vi "Save-Load-Edit ESP Table.vi"(0 "ESP Table Cluster":refnum<vi>, 5 "Table Folder":path, 11 "ESP Table Cluster":T1={"ON-DEMAND Config"=FALSE, "ON-DEMAND Active Commands"=[27, 28, 29], "CONTINUOUS Config"=FALSE, "CONTINUOUS Active Commands"=[41], "ERROR Config"=FALSE, "ERROR Command"="38", "STATUS Config"=FALSE, "STATUS Command"="37", "DIGITAL Config"=FALSE, "DIGITAL Command"="39", "SAVE TABLE"=FALSE, "Active Table"=0, "New Table Name"="38", "NEW CMD TABLE"=[36]} {"Active Table" items=["123", "a", "b", "c"]}, 12 "ENABLE":bool=TRUE) -> (15 "Error Output":errorcluster)   [LabVIEW 2011]
panel:
  # "SAVE - LOAD - EDIT \nESP Command Table"
  # "Blake Otting - Ecolab\nCreated 7-11-2012"
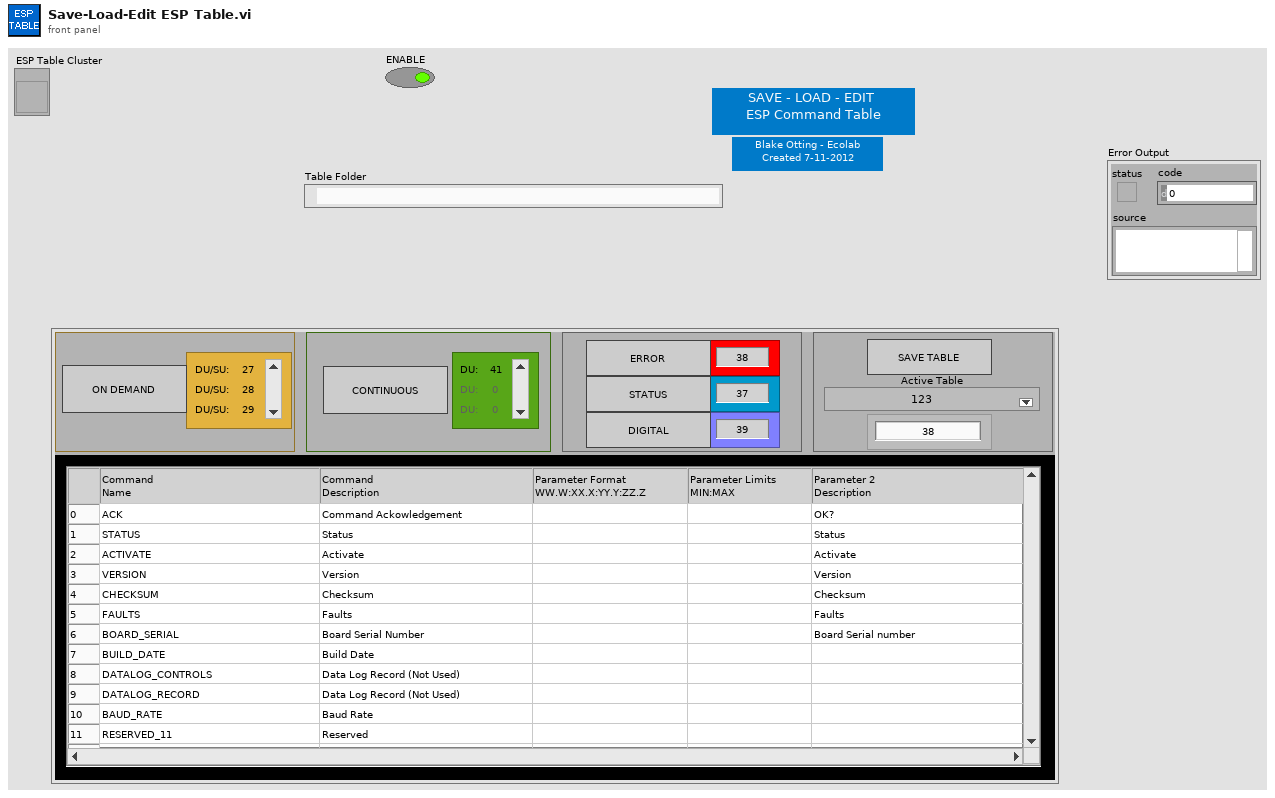
[diagram p1: front panel]
types:
  T1 = cluster{"ON-DEMAND Config":bool, "ON-DEMAND Active Commands":i32[], "CONTINUOUS Config":bool, "CONTINUOUS Active Commands":i32[], "ERROR Config":bool, "ERROR Command":string, "STATUS Config":bool, "STATUS Command":string, "DIGITAL Config":bool, "DIGITAL Command":string, "SAVE TABLE":bool, "Active Table":u16, "New Table Name":string, "NEW CMD TABLE":i32[]}
  T2 = cluster{"ON Demand Button":i32, "ON Demand Commands":i32, "Continuous Button":i32, "Continuous Commands":i32, "Error Button":i32, "Error Command":i32, "Status Button":i32, "Status Command":i32, "Digital Button":i32, "Digital Command":i32, "Save Table Button":i32, "Active Table":i32, "New Table Name":i32, "Table":i32}
  T3 = enum8{"Enabled", "Disabled", "Disabled and Grayed Out"}
  T4 = enum16{"open", "replace", "create", "open or create", "replace or create", "replace or create with confirmation"}
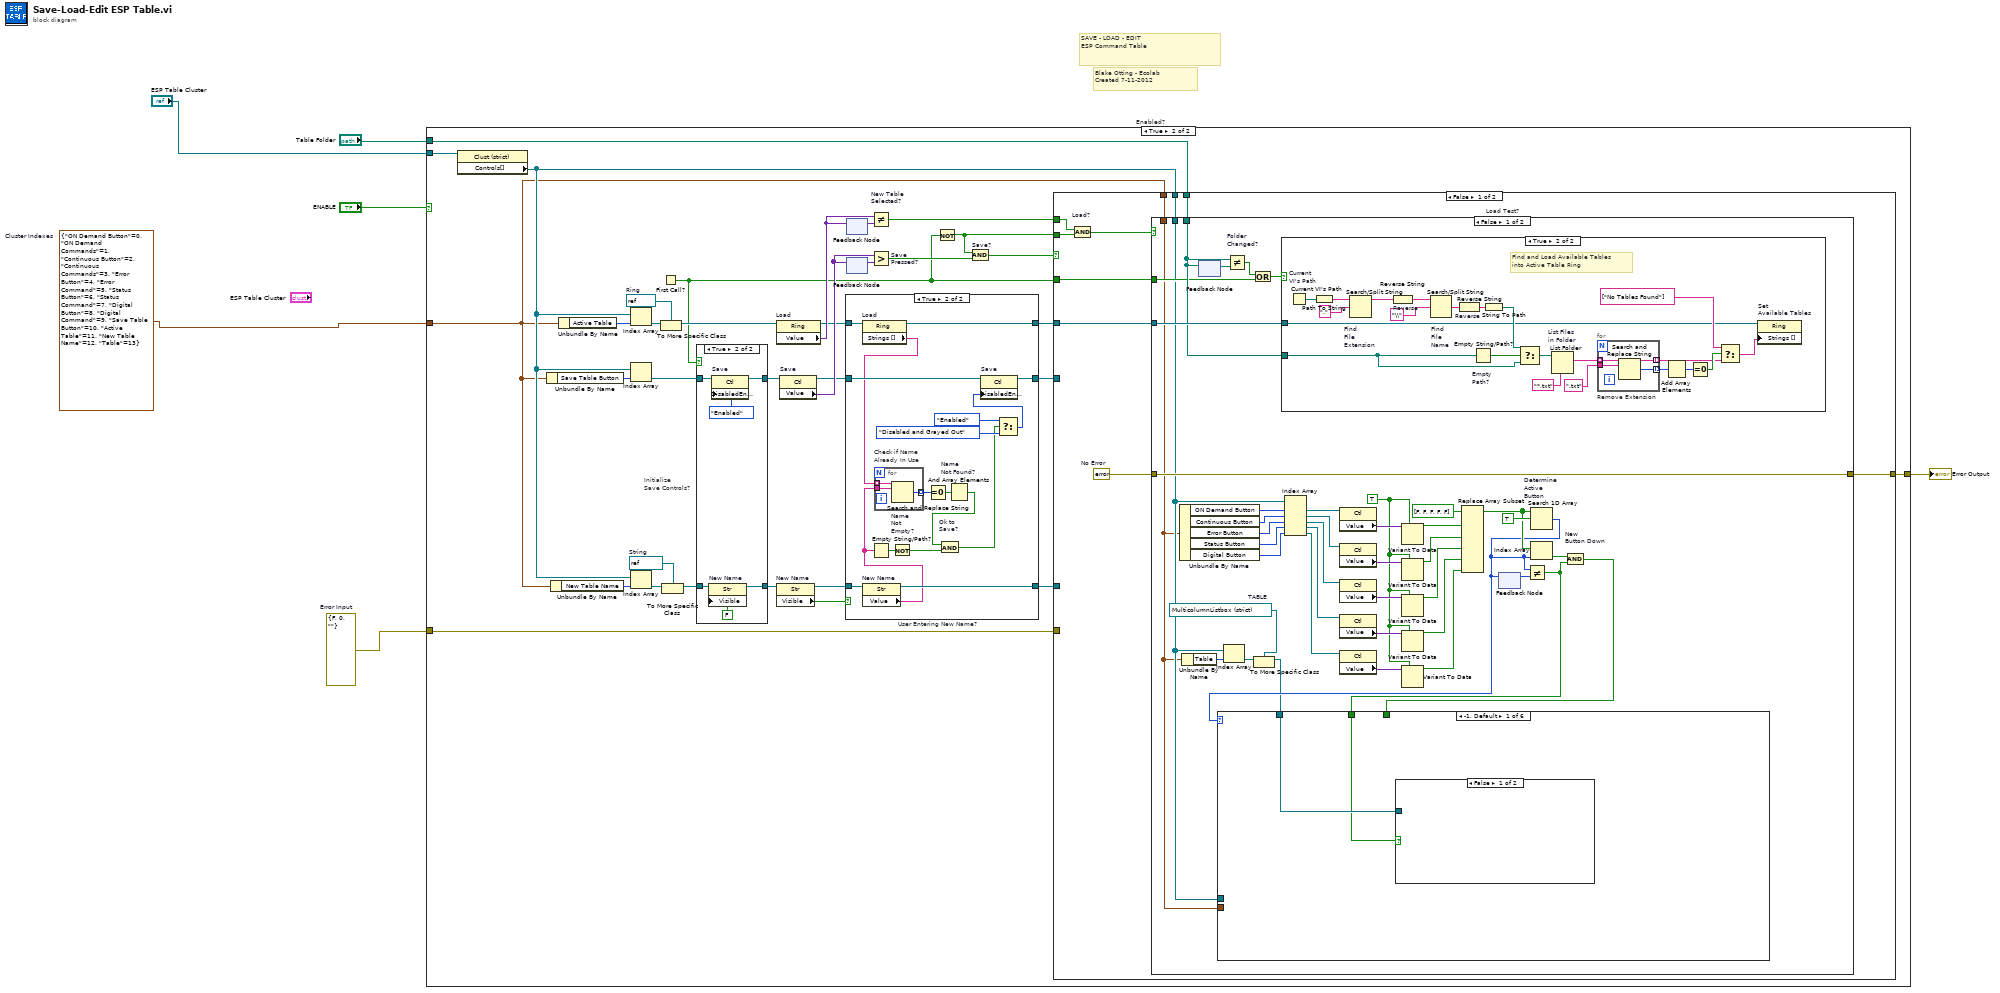
[diagram p0: block diagram]
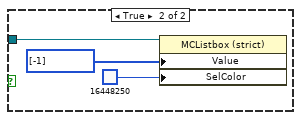
[diagram p5: hidden frame]
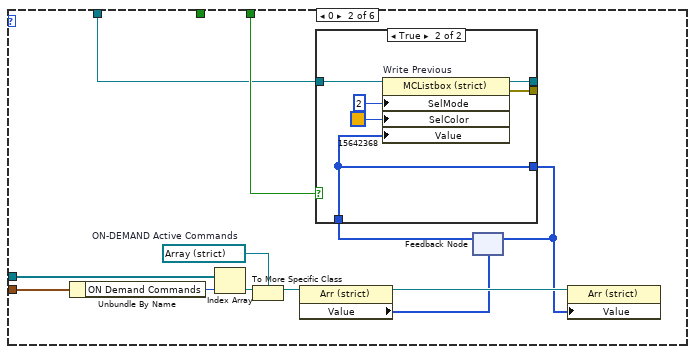
[diagram p6: hidden frame]
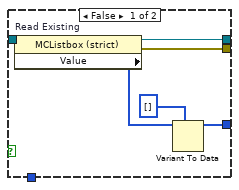
[diagram p7: hidden frame]
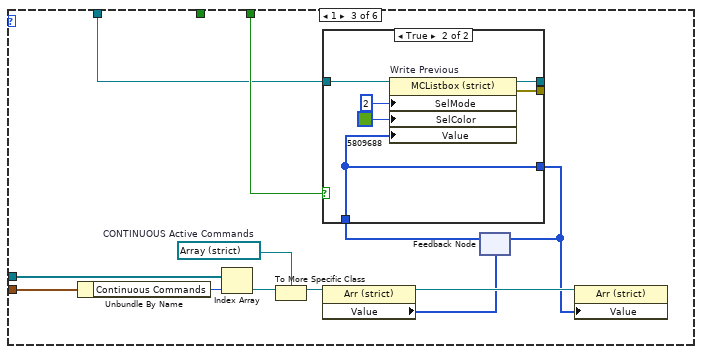
[diagram p8: hidden frame]
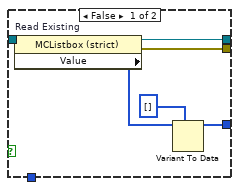
[diagram p9: hidden frame]
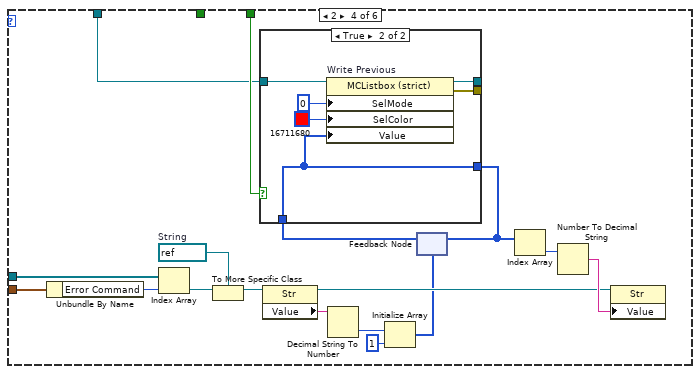
[diagram p10: hidden frame]
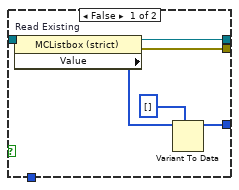
[diagram p11: hidden frame]
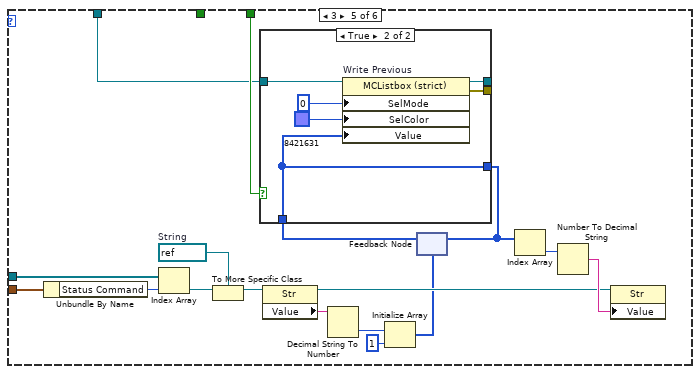
[diagram p12: hidden frame]
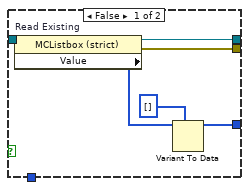
[diagram p13: hidden frame]
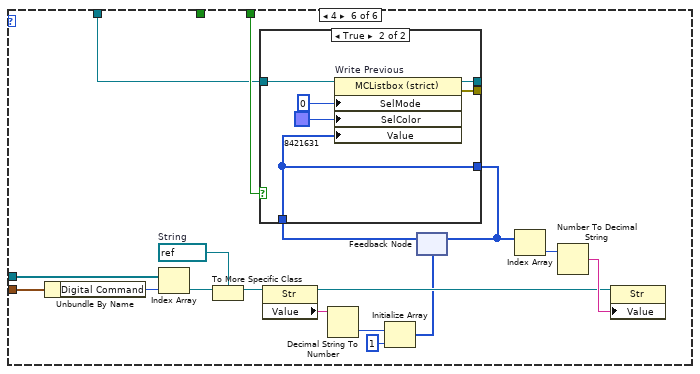
[diagram p14: hidden frame]
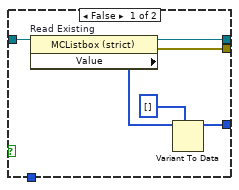
[diagram p15: hidden frame]
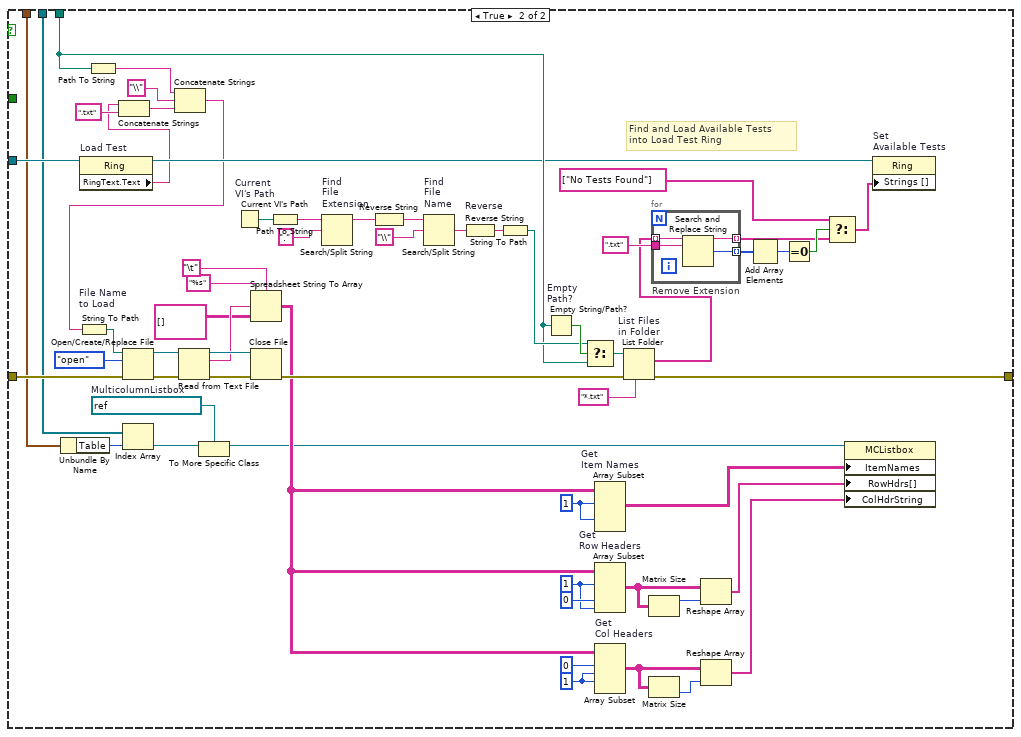
[diagram p17: hidden frame]
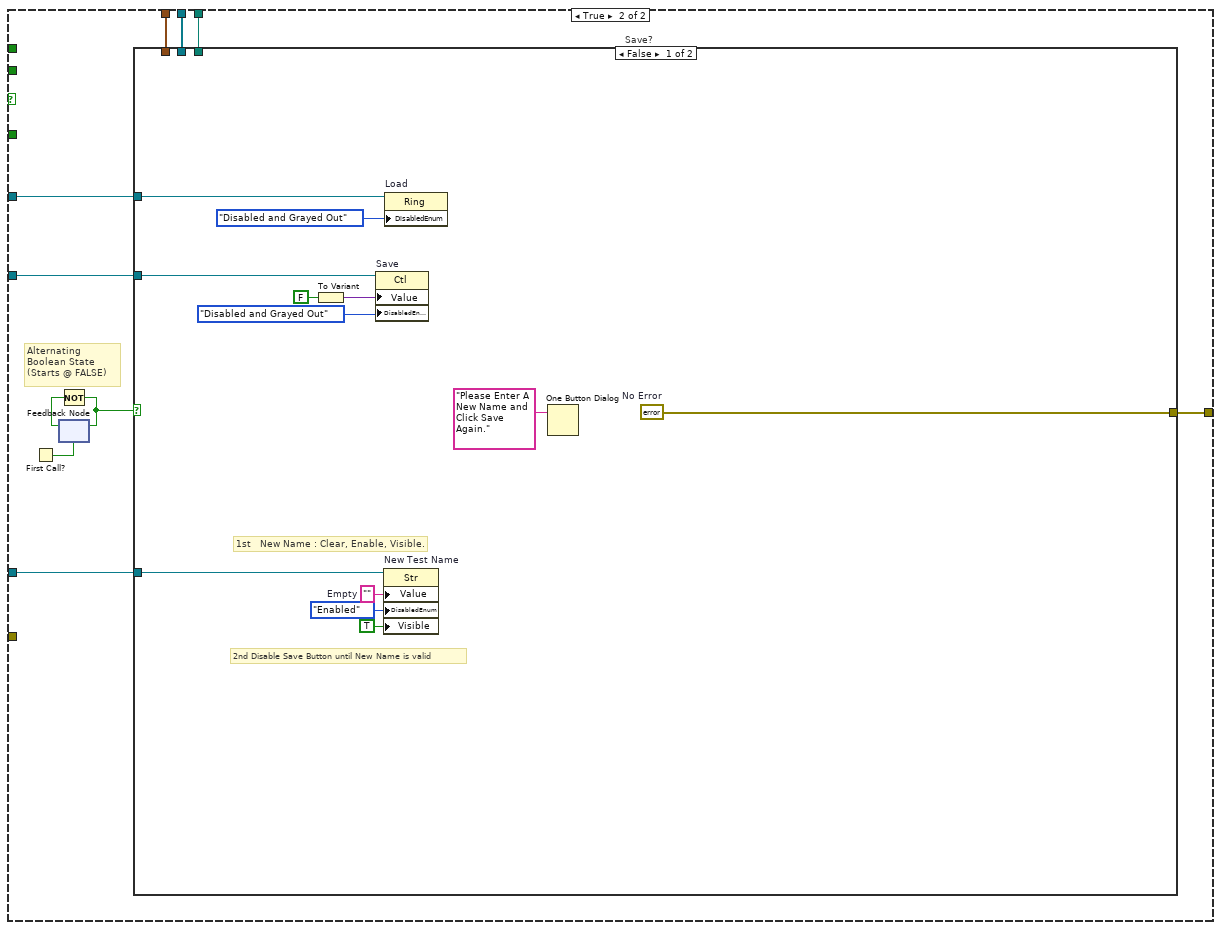
[diagram p18: hidden frame]
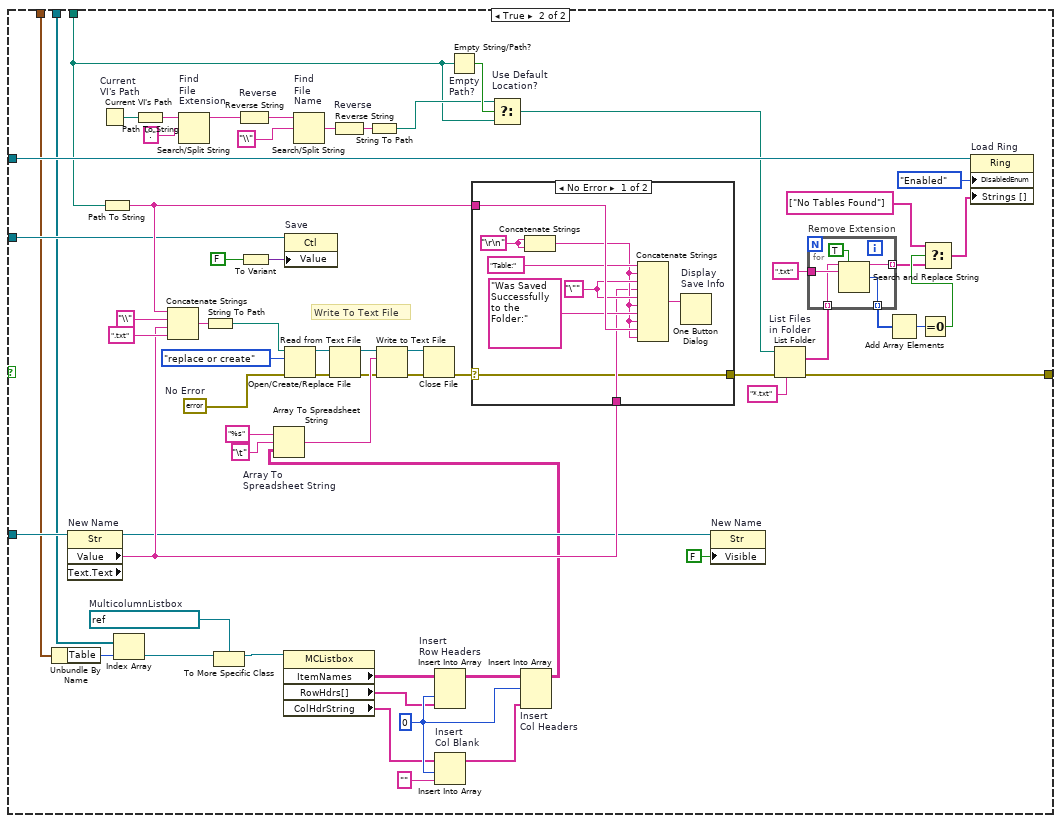
[diagram p19: hidden frame]
diagram:
  w2 = T2 {"ON Demand Button"=0, "ON Demand Commands"=1, "Continuous Button"=2, "Continuous Commands"=3, "Error Button"=4, "Error Command"=5, "Status Button"=6, "Status Command"=7, "Digital Button"=8, "Digital Command"=9, "Save Table Button"=10, "Active Table"=11, "New Table Name"=12, "Table"=13}  # Cluster Indexes
  w3 = errorcluster {"status"=FALSE, "code"=0, "source"=""}  # Error Input
  # "Blake Otting - Ecolab\nCreated 7-11-2012"
  # "SAVE - LOAD - EDIT \nESP Command Table"
  n1 = case "Enabled?" shown="True" "ENABLE" {
    tunnel: "Table Folder" -> [_ w18]
    tunnel: "ESP Table Cluster" -> [_ w13]
    tunnel: [w7 w11] -> w4
    tunnel: w3 -> [w7 w10]
    tunnel: w2 -> [_ w9]
    frame False {
    }
    frame True {
      w22 = refnum<vi> refnum  # Ring
      w40 = refnum<vi> refnum  # String
      n2 = property class="Clust (strict)"(reference=w13) -> ("Controls[]"=w12:refnum<vi>[])  [unwired: 1 in, 2 out]
      n3 = Unbundle By Name(w9) -> ("Save Table Button"=w15:i32)
      n4 = Unbundle By Name(w9) -> ("New Table Name"=w14:i32)
      n5 = Unbundle By Name(w9) -> ("Active Table"=w16:i32)
      n6 = Index Array(array=w12, index=w16) -> (element=w21:refnum<vi>)
      n7 = Index Array(array=w12, index=w15) -> (element=w8:refnum<vi>)
      n8 = Index Array(array=w12, index=w14) -> (element=w41:refnum<vi>)
      n9 = First Call?() -> (First Call?: T/F=w19:bool)
      n10 = To More Specific Class(target class=w22, reference=w21) -> (specific class reference=w20:refnum<vi>)  [unwired: 1 in, 1 out]
      n11 = To More Specific Class(target class=w40, reference=w41) -> (specific class reference=w31:refnum<vi>)  [unwired: 1 in, 1 out]
      n12 = case "Initialize\nSave Controls?" shown="True" w19 {
        tunnel: w8 -> [w42 w49]
        tunnel: [w42 w48] -> w29
        tunnel: w31 -> [w43 w47]
        tunnel: [w43 w46] -> w30
        frame False {
        }
        frame True {
          n13 = property on="New Name" class="Str"(reference=w47, "Visible"=FALSE) -> (reference out=w46:refnum<vi>)  [unwired: 1 in, 1 out]
          n14 = property on="Save" class="Ctl"(reference=w49, "DisabledEnum"=T3."Enabled" ("Disabled")) -> (reference out=w48:refnum<vi>)  [unwired: 1 in, 1 out]
        }
      }
      n15 = property on="Load" class="Ring"(reference=w20) -> (reference out=w25:refnum<vi>, "Value"=w26:variant)  [unwired: 1 in, 1 out]
      n16 = property on="New Name" class="Str"(reference=w30) -> (reference out=w36:refnum<vi>, "Visible"=w37:bool)  [unwired: 1 in, 1 out]
      n17 = property on="Save" class="Ctl"(reference=w29) -> (reference out=w34:refnum<vi>, "Value"=w38:variant)  [unwired: 1 in, 1 out]
      n18 = case "User Entering New Name?" shown="True" w37 {
        tunnel: w36 -> [w52 w65]
        tunnel: w25 -> [w51 w64]
        tunnel: [w52 w60] -> w33
        tunnel: [w51 w59] -> w35
        tunnel: w34 -> [w50 w58]
        tunnel: [w50 w57] -> w32
        frame False {
        }
        frame True {
          n19 = property on="Load" class="Ring"(reference=w64) -> (reference out=w59:refnum<vi>, "Strings []"=w54:string[])  [unwired: 1 in, 1 out]
          n20 = property on="New Name" class="Str"(reference=w65) -> (reference out=w60:refnum<vi>, "Value"=w53:string)  [unwired: 1 in, 1 out]
          n21 = Empty String/Path?(string/path=w53) -> (empty?=w66:bool)
          n22 = for "Check if Name\nAlready In Use" {
            tunnel: w54 -> [w72] mode=indexing
            tunnel: w53 -> [w71]
            tunnel: [w70] -> w69 mode=indexing
            n23 = Search and Replace String(input string=w72, search string=w71) -> (number of replacements=w70:i32)  [unwired: 6 in, 3 out]
          }
          n24 = Not "Name\nNot\nEmpty?"(x=w66) -> (.not. x?=w61:bool)
          n25 = Equal To 0?(x=w69) -> (x = 0?=w68:bool[])
          n26 = And Array Elements "Name\nNot Found?"(Boolean array=w68) -> (logical AND=w67:bool)
          n27 = And "Ok to\nSave?"(x=w67, y=w61) -> (x .and. y?=w55:bool)
          n28 = Select(t=T3."Enabled" ("Disabled"), s=w55, f=T3."Disabled and Grayed Out" ("Disabled")) -> (s? t:f=w56:T3)
          n29 = property on="Save" class="Ctl"(reference=w58, "DisabledEnum"=w56) -> (reference out=w57:refnum<vi>)  [unwired: 1 in, 1 out]
        }
      }
      n30 = feedback #1() -> (w27:variant)  [unwired: 1 in]
      n31 = feedback-in #1(w26) -> ()
      n32 = feedback #2() -> (w39:variant)  [unwired: 1 in]
      n33 = feedback-in #2(w38) -> ()
      n34 = Not Equal? "New Table\nSelected?"(x=w26, y=w27) -> (x != y?=w17:bool)
      n35 = Greater? "Save\nPressed?"(x=w38, y=w39) -> (0:w24:bool)
      n36 = Not(x=w19) -> (.not. x?=w23:bool)
      n37 = And "Save?"(x=w23, y=w24) -> (x .and. y?=w28:bool)
      n38 = case shown="False" w28 {
        tunnel: w18 -> [w79 w357]
        tunnel: w9 -> [w81 w361]
        tunnel: w12 -> [w82 w362]
        tunnel: w32 -> [_ w360]
        tunnel: w33 -> [_ w359]
        tunnel: w35 -> [w80 w358]
        tunnel: [w74 w356] -> w11
        tunnel: w10 -> [_ _]
        tunnel: w17 -> [w76 _]
        tunnel: w19 -> [w78 _]
        tunnel: w23 -> [w75 _]
        frame False {
          w73 = errorcluster {"status"=FALSE, "code"=0, "source"=""}  # No Error
          n39 = And "Load?"(x=w76, y=w75) -> (x .and. y?=w77:bool)
          n40 = case "Load Test?" shown="False" w77 {
            tunnel: w82 -> [w88 w292]
            tunnel: w81 -> [w87 w293]
            tunnel: [w124 w317] -> w74
            tunnel: w73 -> [w124 w311]
            tunnel: w80 -> [w123 w315]
            tunnel: w78 -> [w119 _]
            tunnel: w79 -> [w121 w316]
            frame False {
              w84 = refnum<vi> refnum  # TABLE
              w105 = TRUE
              n41 = Unbundle By Name(w87) -> ("ON Demand Button"=w112:i32, "Continuous Button"=w104:i32, "Error Button"=w103:i32, "Status Button"=w102:i32, "Digital Button"=w101:i32)
              n42 = Unbundle By Name(w87) -> ("Table"=w89:i32)
              n43 = feedback #3() -> (w122:path)  [unwired: 1 in]
              n44 = feedback-in #3(w121) -> ()
              n45 = Index Array(array=w88, index=w89) -> (element=w85:refnum<vi>)
              n46 = Not Equal? "Folder\nChanged?"(x=w121, y=w122) -> (x != y?=w120:bool)
              n47 = Or(x=w120, y=w119) -> (x .or. y?=w118:bool)
              n48 = To More Specific Class(target class=w84, reference=w85) -> (specific class reference=w86:refnum<vi>)  [unwired: 1 in, 1 out]
              n49 = case shown="True" w118 {
                tunnel: w123 -> [_ w266]
                tunnel: w121 -> [_ w265]
                frame False {
                }
                frame True {
                  # "Find and Load Available Tables \ninto Active Table Ring"
                  n50 = Current VI's Path "Current\nVI's Path"() -> (path=w276:path)
                  n51 = Path To String(path=w276) -> (string=w281:string)
                  n52 = Search/Split String "Find\nFile \nExtension"(string=w281, search string/char (-)=".") -> (substring before match=w280:string)  [unwired: 1 in, 2 out]
                  n53 = Reverse String "Reverse"(1:w280) -> (0:w279:string)
                  n54 = Search/Split String "Find\nFile \nName"(string=w279, search string/char (-)="\\") -> (match + rest of string=w277:string)  [unwired: 1 in, 2 out]
                  n55 = Reverse String "Reverse"(1:w277) -> (0:w283:string)
                  n56 = Empty String/Path? "Empty\nPath?"(string/path=w265) -> (empty?=w275:bool)
                  n57 = String To Path(string=w283) -> (path=w274:path)
                  n58 = Select(t=w274, s=w275, f=w265) -> (s? t:f=w284:path)
                  n59 = List Folder "List Files\nin Folder"(path=w284, pattern="*.txt") -> (filenames=w286:string[])  [unwired: 1 in, 4 out]
                  n60 = for "Remove Extension" {
                    tunnel: w286 -> [w289] mode=indexing
                    tunnel: ".txt" ("pattern") -> [w290]
                    tunnel: [w288] -> w267 mode=indexing
                    tunnel: [w287] -> w272 mode=indexing
                    n61 = Search and Replace String(input string=w289, search string=w290) -> (result string=w288:string, number of replacements=w287:i32)  [unwired: 6 in, 2 out]
                  }
                  n62 = Add Array Elements(numeric array=w272) -> (sum=w271:i32)
                  n63 = Equal To 0?(x=w271) -> (x = 0?=w270:bool)
                  n64 = Select(t=string[] ["No Tables Found"], s=w270, f=w267) -> (s? t:f=w269:string[])
                  n65 = property on="Set\nAvailable Tables" class="Ring"(reference=w266, "Strings []"=w269) -> ()  [unwired: 1 in, 2 out]
                }
              }
              n66 = Index Array(array=w88, index #1=w112, index #2=w104, index #3=w103, index #4=w102, index #5=w101) -> (element #1=w100:refnum<vi>, element #2=w99:refnum<vi>, element #3=w98:refnum<vi>, element #4=w96:refnum<vi>, element #5=w97:refnum<vi>)
              n67 = property class="Ctl"(reference=w100) -> ("Value"=w111:variant)  [unwired: 1 in, 2 out]
              n68 = property class="Ctl"(reference=w99) -> ("Value"=w109:variant)  [unwired: 1 in, 2 out]
              n69 = property class="Ctl"(reference=w98) -> ("Value"=w108:variant)  [unwired: 1 in, 2 out]
              n70 = property class="Ctl"(reference=w96) -> ("Value"=w107:variant)  [unwired: 1 in, 2 out]
              n71 = property class="Ctl"(reference=w97) -> ("Value"=w106:variant)  [unwired: 1 in, 2 out]
              n72 = Variant To Data(type=w105, Variant=w111) -> (data=w110:bool)  [unwired: 1 in, 1 out]
              n73 = Variant To Data(type=w105, Variant=w109) -> (data=w95:bool)  [unwired: 1 in, 1 out]
              n74 = Variant To Data(type=w105, Variant=w108) -> (data=w94:bool)  [unwired: 1 in, 1 out]
              n75 = Variant To Data(type=w105, Variant=w107) -> (data=w93:bool)  [unwired: 1 in, 1 out]
              n76 = Variant To Data(type=w105, Variant=w106) -> (data=w92:bool)  [unwired: 1 in, 1 out]
              n77 = Replace Array Subset(array=bool[] [FALSE, FALSE, FALSE, FALSE, FALSE], new element #1=w110, new element #2=w95, new element #3=w94, new element #4=w93, new element #5=w92) -> (w114:bool[])  [unwired: 5 in]
              n78 = feedback #4() -> (w115:i32)  [unwired: 1 in]
              n79 = Search 1D Array "Determine\nActive\nButton"(1D array=w114, element=TRUE) -> (index of element=w90:i32)  [unwired: 1 in]
              n80 = feedback-in #4(w90) -> ()
              n81 = Not Equal?(x=w90, y=w115) -> (x != y?=w83:bool)
              n82 = Index Array(array=w114, index=w90) -> (element=w113:bool)
              n83 = And "New\nButton Down"(x=w113, y=w83) -> (x .and. y?=w91:bool)
              n84 = case shown="-1, Default" w90 {
                tunnel: w91 -> [_ w139 w163 w185 w214 w243]
                tunnel: w87 -> [_ w138 w162 w184 w213 w242]
                tunnel: w88 -> [_ w137 w161 w183 w212 w241]
                tunnel: w86 -> [w126 w133 w157 w178 w207 w236]
                tunnel: w83 -> [w125 _ _ _ _ _]
                frame -1, Default {
                  n85 = case shown="False" w125 {
                    tunnel: w126 -> [_ w129]
                    frame False {
                    }
                    frame True {
                      n86 = property class="MCListbox (strict)"(reference=w129, "Value"=i32[] [-1], "SelColor"=u32 16448250) -> ()  [unwired: 1 in, 2 out]
                    }
                  }
                }
                frame 0 {
                  w132 = refnum<vi> refnum  # ON-DEMAND Active Commands
                  n87 = Unbundle By Name(w138) -> ("ON Demand Commands"=w136:i32)
                  n88 = Index Array(array=w137, index=w136) -> (element=w135:refnum<vi>)
                  n89 = To More Specific Class(target class=w132, reference=w135) -> (specific class reference=w134:refnum<vi>)  [unwired: 1 in, 1 out]
                  n90 = property class="Arr (strict)"(reference=w134) -> (reference out=w140:refnum<vi>, "Value"=w130:i32[])  [unwired: 1 in, 1 out]
                  n91 = feedback #5(w130) -> (w141:i32[])
                  n92 = case shown="True" w139 {
                    tunnel: w133 -> [w147 w153]
                    tunnel: [w142 w148] -> w131
                    tunnel: w141 -> [_ w148]
                    tunnel: [w145 w152] -> _
                    tunnel: [w146 w151] -> _
                    frame False {
                      n93 = property on="Read Existing" class="MCListbox (strict)"(reference=w147) -> (reference out=w145:refnum<vi>, error out=w146:errorcluster, "Value"=w143:i32[])  [unwired: 1 in]
                      n94 = Variant To Data(type=i32[] [], Variant=w143) -> (data=w142:i32[])  [unwired: 1 in, 1 out]
                    }
                    frame True {
                      n95 = property on="Write Previous" class="MCListbox (strict)"(reference=w153, "SelMode"=2, "SelColor"=u32 15642368, "Value"=w148) -> (reference out=w152:refnum<vi>, error out=w151:errorcluster)  [unwired: 1 in]
                    }
                  }
                  n96 = feedback-in #5(w131) -> ()
                  n97 = property class="Arr (strict)"(reference=w140, "Value"=w131) -> ()  [unwired: 1 in, 2 out]
                }
                frame 1 {
                  w156 = refnum<vi> refnum  # CONTINUOUS Active Commands
                  n98 = Unbundle By Name(w162) -> ("Continuous Commands"=w160:i32)
                  n99 = Index Array(array=w161, index=w160) -> (element=w159:refnum<vi>)
                  n100 = To More Specific Class(target class=w156, reference=w159) -> (specific class reference=w158:refnum<vi>)  [unwired: 1 in, 1 out]
                  n101 = property class="Arr (strict)"(reference=w158) -> (reference out=w164:refnum<vi>, "Value"=w154:i32[])  [unwired: 1 in, 1 out]
                  n102 = feedback #6(w154) -> (w165:i32[])
                  n103 = case shown="True" w163 {
                    tunnel: w157 -> [w171 w177]
                    tunnel: [w166 w172] -> w155
                    tunnel: w165 -> [_ w172]
                    tunnel: [w169 w176] -> _
                    tunnel: [w170 w175] -> _
                    frame False {
                      n104 = property on="Read Existing" class="MCListbox (strict)"(reference=w171) -> (reference out=w169:refnum<vi>, error out=w170:errorcluster, "Value"=w167:i32[])  [unwired: 1 in]
                      n105 = Variant To Data(type=i32[] [], Variant=w167) -> (data=w166:i32[])  [unwired: 1 in, 1 out]
                    }
                    frame True {
                      n106 = property on="Write Previous" class="MCListbox (strict)"(reference=w177, "SelMode"=2, "SelColor"=u32 5809688, "Value"=w172) -> (reference out=w176:refnum<vi>, error out=w175:errorcluster)  [unwired: 1 in]
                    }
                  }
                  n107 = feedback-in #6(w155) -> ()
                  n108 = property class="Arr (strict)"(reference=w164, "Value"=w155) -> ()  [unwired: 1 in, 2 out]
                }
                frame 2 {
                  w180 = refnum<vi> refnum  # String
                  n109 = Unbundle By Name(w184) -> ("Error Command"=w182:i32)
                  n110 = Index Array(array=w183, index=w182) -> (element=w181:refnum<vi>)
                  n111 = To More Specific Class(target class=w180, reference=w181) -> (specific class reference=w179:refnum<vi>)  [unwired: 1 in, 1 out]
                  n112 = property class="Str"(reference=w179) -> (reference out=w187:refnum<vi>, "Value"=w190:string)  [unwired: 1 in, 1 out]
                  n113 = Decimal String To Number(string=w190) -> (number=w188:i32)  [unwired: 2 in, 1 out]
                  n114 = Initialize Array(w188, 1) -> (w186:i32[])
                  n115 = feedback #7(w186) -> (w194:i32[])
                  n116 = case shown="True" w185 {
                    tunnel: w178 -> [w200 w206]
                    tunnel: [w195 w201] -> w193
                    tunnel: w194 -> [_ w201]
                    tunnel: [w198 w205] -> _
                    tunnel: [w199 w204] -> _
                    frame False {
                      n117 = property on="Read Existing" class="MCListbox (strict)"(reference=w200) -> (reference out=w198:refnum<vi>, error out=w199:errorcluster, "Value"=w196:i32[])  [unwired: 1 in]
                      n118 = Variant To Data(type=i32[] [], Variant=w196) -> (data=w195:i32[])  [unwired: 1 in, 1 out]
                    }
                    frame True {
                      n119 = property on="Write Previous" class="MCListbox (strict)"(reference=w206, "SelMode"=0, "SelColor"=u32 16711680, "Value"=w201) -> (reference out=w205:refnum<vi>, error out=w204:errorcluster)  [unwired: 1 in]
                    }
                  }
                  n120 = feedback-in #7(w193) -> ()
                  n121 = Index Array(array=w193) -> (element=w192:i32)  [unwired: 1 in]
                  n122 = Number To Decimal String(number=w192) -> (decimal integer string=w191:string)  [unwired: 1 in]
                  n123 = property class="Str"(reference=w187, "Value"=w191) -> ()  [unwired: 1 in, 2 out]
                }
                frame 3 {
                  w209 = refnum<vi> refnum  # String
                  n124 = Unbundle By Name(w213) -> ("Status Command"=w211:i32)
                  n125 = Index Array(array=w212, index=w211) -> (element=w210:refnum<vi>)
                  n126 = To More Specific Class(target class=w209, reference=w210) -> (specific class reference=w208:refnum<vi>)  [unwired: 1 in, 1 out]
                  n127 = property class="Str"(reference=w208) -> (reference out=w216:refnum<vi>, "Value"=w219:string)  [unwired: 1 in, 1 out]
                  n128 = Decimal String To Number(string=w219) -> (number=w217:i32)  [unwired: 2 in, 1 out]
                  n129 = Initialize Array(w217, 1) -> (w215:i32[])
                  n130 = feedback #8(w215) -> (w223:i32[])
                  n131 = case shown="True" w214 {
                    tunnel: w207 -> [w229 w235]
                    tunnel: [w224 w230] -> w222
                    tunnel: w223 -> [_ w230]
                    tunnel: [w227 w234] -> _
                    tunnel: [w228 w233] -> _
                    frame False {
                      n132 = property on="Read Existing" class="MCListbox (strict)"(reference=w229) -> (reference out=w227:refnum<vi>, error out=w228:errorcluster, "Value"=w225:i32[])  [unwired: 1 in]
                      n133 = Variant To Data(type=i32[] [], Variant=w225) -> (data=w224:i32[])  [unwired: 1 in, 1 out]
                    }
                    frame True {
                      n134 = property on="Write Previous" class="MCListbox (strict)"(reference=w235, "SelMode"=0, "SelColor"=u32 8421631, "Value"=w230) -> (reference out=w234:refnum<vi>, error out=w233:errorcluster)  [unwired: 1 in]
                    }
                  }
                  n135 = feedback-in #8(w222) -> ()
                  n136 = Index Array(array=w222) -> (element=w221:i32)  [unwired: 1 in]
                  n137 = Number To Decimal String(number=w221) -> (decimal integer string=w220:string)  [unwired: 1 in]
                  n138 = property class="Str"(reference=w216, "Value"=w220) -> ()  [unwired: 1 in, 2 out]
                }
                frame 4 {
                  w238 = refnum<vi> refnum  # String
                  n139 = Unbundle By Name(w242) -> ("Digital Command"=w240:i32)
                  n140 = Index Array(array=w241, index=w240) -> (element=w239:refnum<vi>)
                  n141 = To More Specific Class(target class=w238, reference=w239) -> (specific class reference=w237:refnum<vi>)  [unwired: 1 in, 1 out]
                  n142 = property class="Str"(reference=w237) -> (reference out=w245:refnum<vi>, "Value"=w248:string)  [unwired: 1 in, 1 out]
                  n143 = Decimal String To Number(string=w248) -> (number=w246:i32)  [unwired: 2 in, 1 out]
                  n144 = Initialize Array(w246, 1) -> (w244:i32[])
                  n145 = feedback #9(w244) -> (w252:i32[])
                  n146 = case shown="True" w243 {
                    tunnel: w236 -> [w258 w264]
                    tunnel: [w253 w259] -> w251
                    tunnel: w252 -> [_ w259]
                    tunnel: [w256 w263] -> _
                    tunnel: [w257 w262] -> _
                    frame False {
                      n147 = property on="Read Existing" class="MCListbox (strict)"(reference=w258) -> (reference out=w256:refnum<vi>, error out=w257:errorcluster, "Value"=w254:i32[])  [unwired: 1 in]
                      n148 = Variant To Data(type=i32[] [], Variant=w254) -> (data=w253:i32[])  [unwired: 1 in, 1 out]
                    }
                    frame True {
                      n149 = property on="Write Previous" class="MCListbox (strict)"(reference=w264, "SelMode"=0, "SelColor"=u32 8421631, "Value"=w259) -> (reference out=w263:refnum<vi>, error out=w262:errorcluster)  [unwired: 1 in]
                    }
                  }
                  n150 = feedback-in #9(w251) -> ()
                  n151 = Index Array(array=w251) -> (element=w250:i32)  [unwired: 1 in]
                  n152 = Number To Decimal String(number=w250) -> (decimal integer string=w249:string)  [unwired: 1 in]
                  n153 = property class="Str"(reference=w245, "Value"=w249) -> ()  [unwired: 1 in, 2 out]
                }
              }
            }
            frame True {
              w295 = refnum<vi> refnum  # MulticolumnListbox
              w304 = 1
              w307 = 1
              w309 = 1
              # "Find and Load Available Tests \ninto Load Test Ring"
              n154 = Unbundle By Name(w293) -> ("Table"=w294:i32)
              n155 = property on="Load Test" class="Ring"(reference=w315) -> (reference out=w314:refnum<vi>, "RingText.Text"=w313:string)  [unwired: 1 in, 1 out]
              n156 = Path To String(path=w316) -> (string=w339:string)
              n157 = Concatenate Strings(w313, ".txt" ("string")) -> (w341:string)
              n158 = Index Array(array=w292, index=w294) -> (element=w296:refnum<vi>)
              n159 = Concatenate Strings(w339, "\\" ("string"), w341) -> (w312:string)
              n160 = String To Path "File Name\nto Load"(string=w312) -> (path=w348:path)
              n161 = Open/Create/Replace File(file path (use dialog)=w348, error in=w311, operation (0:open)=T4."open") -> (refnum out=w350:refnum<file>, error out=w343:errorcluster)  [unwired: 3 in, 1 out]
              n162 = Read from Text File(file (use dialog)=w350, error in=w343) -> (refnum out=w351:refnum<file>, text=w349:string, error out=w342:errorcluster)  [unwired: 3 out]
              n163 = To More Specific Class(target class=w295, reference=w296) -> (specific class reference=w291:refnum<vi>)  [unwired: 1 in, 1 out]
              n164 = Current VI's Path "Current\nVI's Path"() -> (path=w328:path)
              n165 = Spreadsheet String To Array(delimiter (Tab)="\t" ("delimiter (\\t)"), format string="%s" ("format (%s)"), spreadsheet string=w349, array type (2D Dbl)=string[][] [] ("appended array")) -> (array=w297:string[][])
              n166 = Close File(refnum=w351, error in=w342) -> (error out=w318:errorcluster)  [unwired: 1 out]
              n167 = Path To String(path=w328) -> (string=w333:string)
              n168 = Search/Split String "Find\nFile \nExtension"(string=w333, search string/char (-)=".") -> (substring before match=w332:string)  [unwired: 1 in, 2 out]
              n169 = Reverse String(1:w332) -> (0:w331:string)
              n170 = Search/Split String "Find\nFile \nName"(string=w331, search string/char (-)="\\") -> (match + rest of string=w329:string)  [unwired: 1 in, 2 out]
              n171 = Reverse String "Reverse"(1:w329) -> (0:w335:string)
              n172 = String To Path(string=w335) -> (path=w326:path)
              n173 = Empty String/Path? "Empty\nPath?"(string/path=w316) -> (empty?=w327:bool)
              n174 = Select(t=w326, s=w327, f=w316) -> (s? t:f=w336:path)
              n175 = Array Subset "Get\nItem Names"(array=w297, index (row)=w309, index (col)=w309) -> (w300:string[][])  [unwired: 2 in]
              n176 = Array Subset "Get\nRow Headers"(array=w297, index (row)=w307, index (col)=0, length (col)=w307) -> (w303:string[][])  [unwired: 1 in]
              n177 = Array Subset "Get\nCol Headers"(array=w297, index (row)=0, length (row)=w304, index (col)=w304) -> (w302:string[][])  [unwired: 1 in]
              n178 = List Folder "List Files\nin Folder"(path=w336, pattern="*.txt", error in=w318) -> (filenames=w310:string[], error out=w317:errorcluster)  [unwired: 3 out]
              n179 = Matrix Size(0:w303) -> (1:w306:i32)  [unwired: 1 out]
              n180 = Matrix Size(0:w302) -> (2:w301:i32)  [unwired: 1 out]
              n181 = for "Remove Extension" {
                tunnel: w310 -> [w354] mode=indexing
                tunnel: ".txt" ("pattern") -> [w355]
                tunnel: [w353] -> w319 mode=indexing
                tunnel: [w352] -> w324 mode=indexing
                n182 = Search and Replace String(input string=w354, search string=w355) -> (result string=w353:string, number of replacements=w352:i32)  [unwired: 6 in, 2 out]
              }
              n183 = Reshape Array(w303, w306) -> (w299:string[])
              n184 = Reshape Array(w302, w301) -> (w298:string[])
              n185 = Add Array Elements(numeric array=w324) -> (sum=w323:i32)
              n186 = Equal To 0?(x=w323) -> (x = 0?=w322:bool)
              n187 = Select(t=string[] ["No Tests Found"], s=w322, f=w319) -> (s? t:f=w321:string[])
              n188 = property class="MCListbox"(reference=w291, "ItemNames"=w300, "RowHdrs[]"=w299, "ColHdrString"=w298) -> ()  [unwired: 1 in, 2 out]
              n189 = property on="Set\nAvailable Tests" class="Ring"(reference=w314, "Strings []"=w321) -> ()  [unwired: 1 in, 2 out]
            }
          }
        }
        frame True {
          # "Alternating\nBoolean State\n(Starts @ FALSE)"
          n190 = First Call?() -> (First Call?: T/F=w364:bool)
          n191 = feedback #10(w364) -> (w365:bool)
          n192 = Not(x=w365) -> (.not. x?=w363:bool)
          n193 = feedback-in #10(w363) -> ()
          n194 = case "Save?" shown="False" w363 {
            tunnel: w361 -> [_ w381]
            tunnel: w362 -> [_ w380]
            tunnel: w360 -> [w373 w418]
            tunnel: w359 -> [w370 w422]
            tunnel: w358 -> [w369 w417]
            tunnel: w357 -> [_ w394]
            tunnel: [w366 w395] -> w356
            frame False {
              w366 = errorcluster {"status"=FALSE, "code"=0, "source"=""}  # No Error
              w375 = ""  # Empty
              # "2nd Disable Save Button until New Name is valid"
              # "1st   New Name : Clear, Enable, Visible."
              n195 = To Variant(anything=FALSE ("Value")) -> (Variant=w371:variant)
              n196 = property on="Save" class="Ctl"(reference=w373, "Value"=w371, "DisabledEnum"=T3."Disabled and Grayed Out" ("Disabled")) -> ()  [unwired: 1 in, 2 out]
              n197 = property on="New Test Name" class="Str"(reference=w370, "Value"=w375, "DisabledEnum"=T3."Enabled" ("Disabled"), "Visible"=TRUE) -> ()  [unwired: 1 in, 2 out]
              n198 = property on="Load" class="Ring"(reference=w369, "DisabledEnum"=T3."Disabled and Grayed Out" ("Disabled")) -> ()  [unwired: 1 in, 2 out]
              n199 = One Button Dialog(message="Please Enter A New Name and Click Save Again.") -> ()  [unwired: 1 in, 1 out]
            }
            frame True {
              w379 = refnum<vi> refnum  # MulticolumnListbox
              w391 = 0
              w392 = errorcluster {"status"=FALSE, "code"=0, "source"=""}  # No Error
              # "Write To Text File"
              n200 = Unbundle By Name(w381) -> ("Table"=w383:i32)
              n201 = property on="New Name" class="Str" props=["Value", "Text", "Text"](reference=w422) -> (reference out=w421:refnum<vi>, "Value"=w423:string)  [unwired: 1 in, 2 out]
              n202 = Current VI's Path "Current\nVI's Path"() -> (path=w406:path)
              n203 = Path To String(path=w394) -> (string=w426:string)
              n204 = Index Array(array=w380, index=w383) -> (element=w382:refnum<vi>)
              n205 = Path To String(path=w406) -> (string=w411:string)
              n206 = Concatenate Strings(w426, "\\" ("string"), w423, ".txt" ("string")) -> (w438:string)
              n207 = Search/Split String "Find\nFile \nExtension"(string=w411, search string/char (-)=".") -> (substring before match=w410:string)  [unwired: 1 in, 2 out]
              n208 = String To Path(string=w438) -> (path=w434:path)
              n209 = To More Specific Class(target class=w379, reference=w382) -> (specific class reference=w378:refnum<vi>)  [unwired: 1 in, 1 out]
              n210 = Reverse String "Reverse"(1:w410) -> (0:w409:string)
              n211 = To Variant(anything=FALSE ("Value")) -> (Variant=w419:variant)
              n212 = property class="MCListbox"(reference=w378) -> ("ItemNames"=w387:string[][], "RowHdrs[]"=w386:string[], "ColHdrString"=w385:string[])  [unwired: 1 in, 2 out]
              n213 = property on="Save" class="Ctl"(reference=w418, "Value"=w419) -> ()  [unwired: 1 in, 2 out]
              n214 = Open/Create/Replace File(file path (use dialog)=w434, error in=w392, operation (0:open)=T4."replace or create") -> (refnum out=w435:refnum<file>, error out=w437:errorcluster)  [unwired: 3 in, 1 out]
              n215 = Search/Split String "Find\nFile \nName"(string=w409, search string/char (-)="\\") -> (match + rest of string=w407:string)  [unwired: 1 in, 2 out]
              n216 = Read from Text File(file (use dialog)=w435, error in=w437) -> (refnum out=w428:refnum<file>, error out=w427:errorcluster)  [unwired: 4 out]
              n217 = Reverse String "Reverse"(1:w407) -> (0:w413:string)
              n218 = String To Path(string=w413) -> (path=w404:path)
              n219 = Insert Into Array "Insert \nRow Headers"(array=w387, index (col)=w391, new element=w386) -> (w388:string[][])  [unwired: 1 in]
              n220 = Insert Into Array "Insert\nCol Blank"(array=w385, index=w391, new element="") -> (w390:string[])
              n221 = Empty String/Path? "Empty\nPath?"(string/path=w394) -> (empty?=w405:bool)
              n222 = Select "Use Default\nLocation?"(t=w404, s=w405, f=w394) -> (s? t:f=w414:path)
              n223 = Insert Into Array "Insert\nCol Headers"(array=w388, index (row)=w391, new element=w390) -> (w384:string[][])  [unwired: 1 in]
              n224 = Array To Spreadsheet String "Array To \nSpreadsheet String"(delimiter (Tab)="\t" ("delimiter (\\t)"), array=w384, 3:"%s" ("format (%s)")) -> (spreadsheet string=w431:string)
              n225 = Write to Text File ("Write to\nText File")(file (use dialog)=w428, text=w431, error in=w427) -> (refnum out=w430:refnum<file>, error out=w429:errorcluster)  [unwired: 1 in, 1 out]
              n226 = Close File(refnum=w430, error in=w429) -> (error out=w424:errorcluster)  [unwired: 1 out]
              n227 = case shown="No Error" w424 {
                selector: w424 -> [w446 w455]
                tunnel: w426 -> [w454 _]
                tunnel: w423 -> [w447 _]
                tunnel: [w446 w455] -> w396
                frame No Error {
                  w452 = "\r\n"
                  w450 = "\""
                  n228 = Concatenate Strings(w452, w452) -> (w448:string)
                  n229 = Concatenate Strings("Table:", w448, w450, w447, w450, w448, "Was Saved Successfully to the Folder:", w448, w454, w448) -> (w453:string)
                  n230 = One Button Dialog "Display\nSave Info"(message=w453) -> ()  [unwired: 1 in, 1 out]
                }
                frame Error {
                }
              }
              n231 = property on="New Name" class="Str"(reference=w421, "Visible"=FALSE) -> ()  [unwired: 1 in, 2 out]
              n232 = List Folder "List Files\nin Folder"(path=w414, pattern="*.txt", error in=w396) -> (filenames=w416:string[], error out=w395:errorcluster)  [unwired: 3 out]
              n233 = for "Remove Extension" {
                tunnel: w416 -> [w444] mode=indexing
                tunnel: ".txt" ("pattern") -> [w445]
                tunnel: [w443] -> w397 mode=indexing
                tunnel: [w441] -> w402 mode=indexing
                n234 = Search and Replace String(replace all?=TRUE ("replace all? (F)"), input string=w444, search string=w445) -> (result string=w443:string, number of replacements=w441:i32)  [unwired: 5 in, 2 out]
              }
              n235 = Add Array Elements(numeric array=w402) -> (sum=w401:i32)
              n236 = Equal To 0?(x=w401) -> (x = 0?=w400:bool)
              n237 = Select(t=string[] ["No Tables Found"], s=w400, f=w397) -> (s? t:f=w399:string[])
              n238 = property on="Load Ring" class="Ring"(reference=w417, "DisabledEnum"=T3."Enabled" ("Disabled"), "Strings []"=w399) -> ()  [unwired: 1 in, 2 out]
            }
          }
        }
      }
    }
  }
  "Error Output" <- w4
